vi "Analyze.vi"(0 "Analyze BaseClass in":refnum<class "Analyze BaseClass.lvclass">, 1 "Create Overlay?":bool, 5 "Image in":T1, 7 "Parameters":variant, 9 "Results in":variant, 11 "error in (no error)":errorcluster) -> (4 "Analyze BaseClass out":refnum<class "Analyze BaseClass.lvclass">, 6 "Image out":T1, 8 "Parameters out":variant, 10 "Results":variant, 15 "error out":errorcluster)   [LabVIEW 2020, in "Analyze.lvlib" / "Analyze BaseClass.lvclass"]
uses:
  Analyze BaseClass.lvclass
  <vilib>/vision/Image Controls.llb/IMAQ Image.ctl
  Analyze BaseClass.lvclass/Analyze BaseClass.ctl
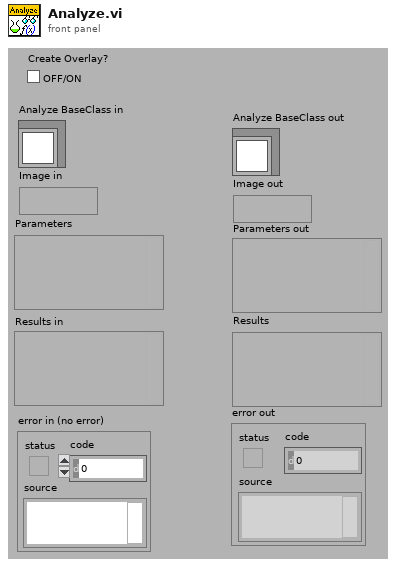
[diagram p1: front panel]
types:
  T1 = typedef "IMAQ Image.ctl" = refnum<image>
  T2 = typedef "ROI Descriptor" = cluster{"Global Rectangle":i32[], "Contours":cluster{"ID":enum32{"External", "Internal"}, "Type":u32, "Coordinates":i32[]}[]}
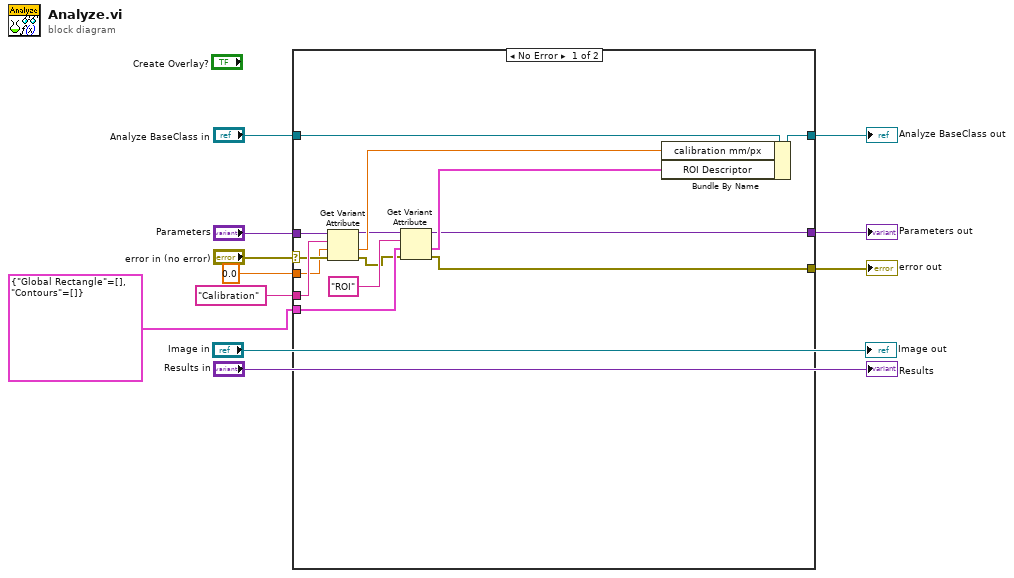
[diagram p0: block diagram]
diagram:
  n1 = case shown="No Error" "error in (no error)" {
    selector: "error in (no error)" -> [w21 w28]
    tunnel: [w13 w28] -> w10
    tunnel: [w24 w27] -> w8
    tunnel: "Analyze BaseClass in" -> [w25 w27]
    tunnel: "Parameters" -> [w23 w26]
    tunnel: "Calibration" ("name") -> [w22 _]
    tunnel: 0.0 -> [w20 _]
    tunnel: T2 {"Global Rectangle"=[], "Contours"=[]} ("ROI") -> [w18 _]
    tunnel: [w12 w26] -> w1
    frame No Error {
      n2 = Get Variant Attribute(Variant=w23, name=w22, default value (empty Variant)=w20, error in=w21) -> (duplicate Variant=w17:variant, value=w19:dbl, error out=w14:errorcluster)  [unwired: 1 out]
      n3 = Get Variant Attribute(Variant=w17, name="ROI", default value (empty Variant)=w18, error in=w14) -> (duplicate Variant=w12:variant, value=w15:T2, error out=w13:errorcluster)  [unwired: 1 out]
      n4 = Bundle By Name(cluster=w25, "calibration mm/px"=w19, "ROI Descriptor"=w15) -> (w24:refnum<class "Analyze BaseClass.lvclass">)
    }
    frame Error {
    }
  }
  "error out" <- w10
  "Analyze BaseClass out" <- w8
  "Parameters out" <- w1
  "Results" <- "Results in"
  "Image out" <- "Image in"
